vi "Hardware Manual Controller.vi"(6 "Simulated":bool, 7 "Simulated Actual Pressure":dbl, 8 "error in (no error)":errorcluster, 9 "Manual Control Cluster":T1 {"Speed" scale=0.0..10.0}, 10 "DAQ Ref Cluster in":T4, 11 "State Machine Data":T2={"Control State"="", "Status Message"="", "Speed"=0.0, "Pressure"=0.0, "Target Pressure"=0.0, "Apply Brake Ref"=refnum, "Release Brake Ref"=refnum, "Extend Ref"=refnum, "Retract Ref"=refnum, "Pressure Ref"=refnum, "Data Display Ref"=refnum, "Exit Button Ref"=refnum, "Bool"=TRUE, "Status"={"Extend"=FALSE, "Brake"=FALSE, "Retract"=FALSE}}) -> (0 "error out":errorcluster, 2 "DAQ Ref Cluster out":T4, 3 "Data Cluster out":T5)   [LabVIEW 2021]
uses:
  Controls/UI Data.ctl
  Controls/Status Lights.ctl
  Controls/DAQ Refnums.ctl
  Controls/State Machine Data.ctl
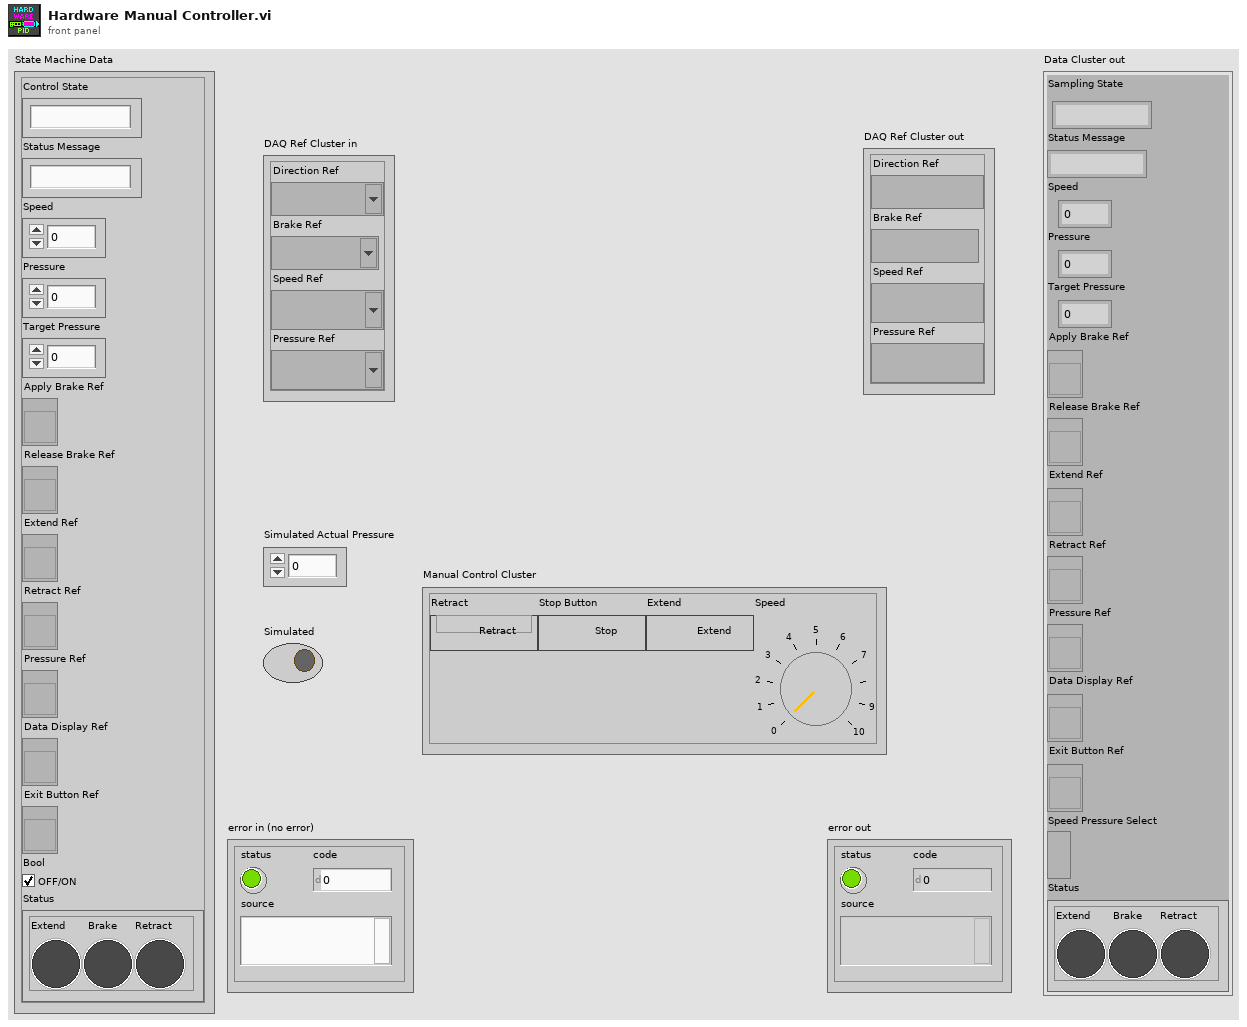
[diagram p1: front panel]
types:
  T1 = cluster{"Retract":bool, "Stop Button":bool, "Extend":bool, "Speed":dbl}
  T2 = typedef "State Machine Data.ctl" = cluster{"Control State":string, "Status Message":string, "Speed":dbl, "Pressure":dbl, "Target Pressure":dbl, "Apply Brake Ref":refnum<vi>, "Release Brake Ref":refnum<vi>, "Extend Ref":refnum<vi>, "Retract Ref":refnum<vi>, "Pressure Ref":refnum<vi>, "Data Display Ref":refnum<vi>, "Exit Button Ref":refnum<vi>, "Bool":bool, "Status":T3}
  T3 = typedef "Status Lights.ctl" = cluster{"Extend":bool, "Brake":bool, "Retract":bool}
  T4 = typedef "DAQ Refnums.ctl" = cluster{"Direction Ref":refnum<k21>, "Brake Ref":refnum<k21>, "Speed Ref":refnum<k21>, "Pressure Ref":refnum<k21>}
  T5 = typedef "UI Data.ctl" = cluster{"Sampling State":string, "Status Message":string, "Speed":dbl, "Pressure":dbl, "Target Pressure":dbl, "Apply Brake Ref":refnum<vi>, "Release Brake Ref":refnum<vi>, "Extend Ref":refnum<vi>, "Retract Ref":refnum<vi>, "Pressure Ref":refnum<vi>, "Data Display Ref":refnum<vi>, "Exit Button Ref":refnum<vi>, "Speed Pressure Select":bool, "Status":T3}
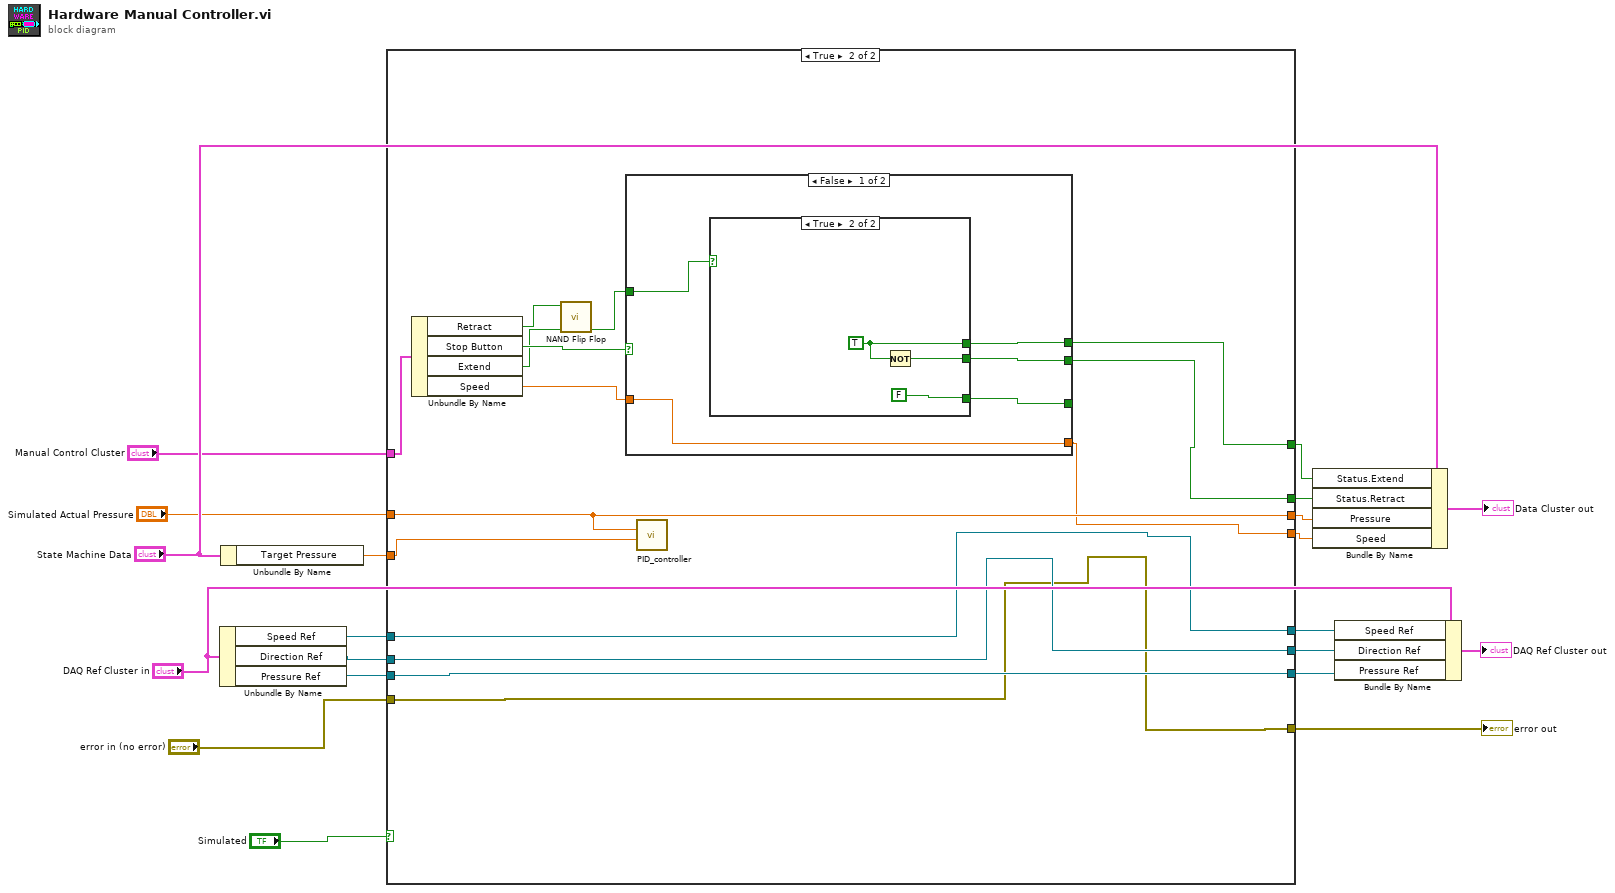
[diagram p0: block diagram]
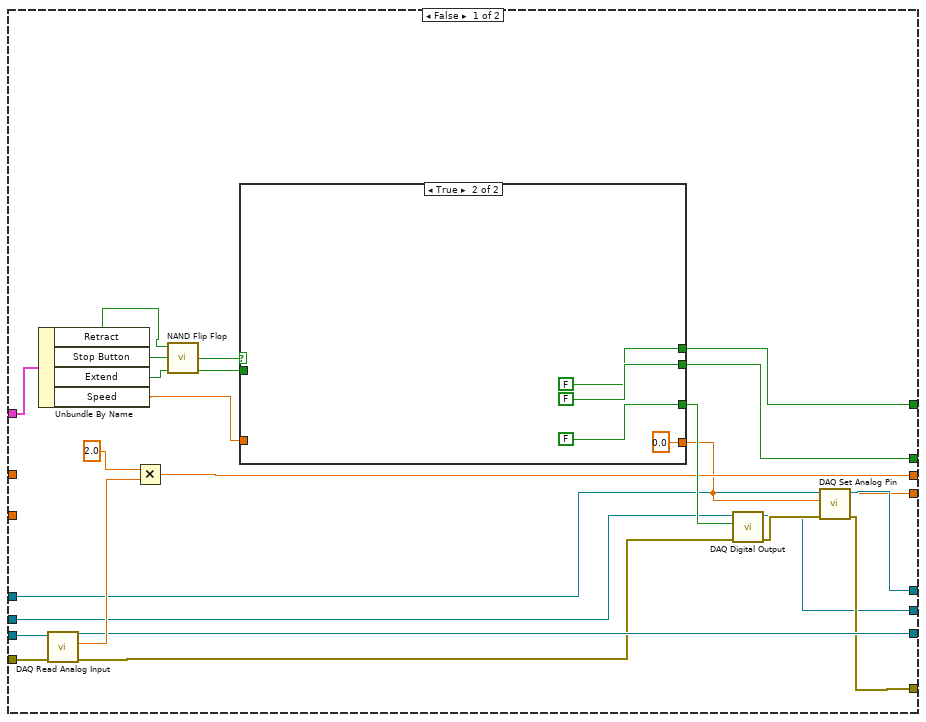
[diagram p2: hidden frame]
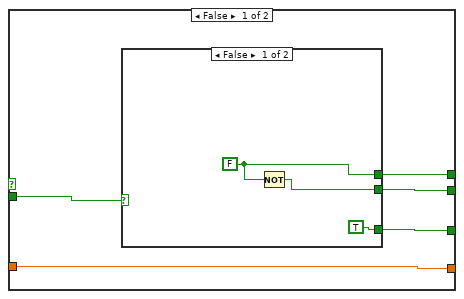
[diagram p3: hidden frame]
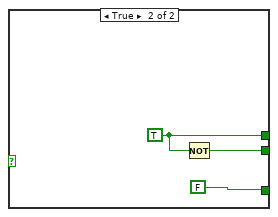
[diagram p4: hidden frame]
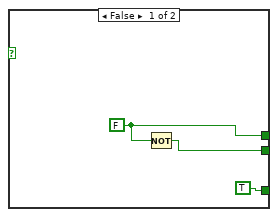
[diagram p5: hidden frame]
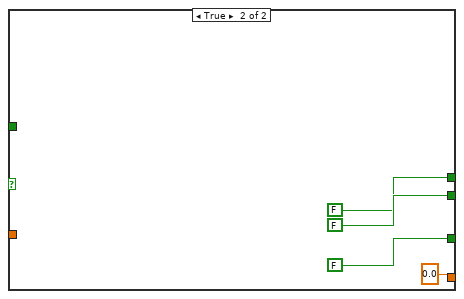
[diagram p6: hidden frame]
diagram:
  n1 = Unbundle By Name("DAQ Ref Cluster in") -> ("Speed Ref"=w10:refnum<k21>, "Direction Ref"=w12:refnum<k21>, "Pressure Ref"=w14:refnum<k21>)
  n2 = Unbundle By Name("State Machine Data") -> ("Target Pressure"=w20:dbl)
  n3 = case shown="True" "Simulated" {
    tunnel: w20 -> [_ w73]
    tunnel: "error in (no error)" -> [w43 w68]
    tunnel: [w41 w72] -> w18
    tunnel: w14 -> [w40 w72]
    tunnel: [w36 w68] -> w13
    tunnel: w12 -> [w35 w70]
    tunnel: [w34 w70] -> w11
    tunnel: w10 -> [w33 w69]
    tunnel: [w32 w69] -> w9
    tunnel: [w21 w61] -> w8
    tunnel: [w28 w71] -> w7
    tunnel: [w30 w67] -> w5
    tunnel: [w29 w66] -> w4
    tunnel: "Simulated Actual Pressure" -> [_ w71]
    tunnel: "Manual Control Cluster" -> [w27 w64]
    frame False {
      n4 = Unbundle By Name(w27) -> ("Retract"=w24:bool, "Stop Button"=w26:bool, "Extend"=w25:bool, "Speed"=w22:dbl)
      n5 = call "DAQ Read Analog Input.vi"("error in"=w43, "task/channels in"=w40) -> ("error out"=w38:errorcluster, "Voltage"=w42:dbl, "task out"=w41:refnum<k21>)  [unwired: 7 in]
      n6 = Multiply(x=2.0, y=w42) -> (x*y=w28:dbl)
      n7 = call "NAND Flip Flop.vi"("Reset"=w25, "Set"=w24) -> ("!Q"=w23:bool)  [unwired: 8 in, 1 out]
      n8 = case shown="True" w26 {
        tunnel: [w48 FALSE ("data")] -> w39
        tunnel: [w47 FALSE ("Status.Extend")] -> w30
        tunnel: [w46 FALSE] -> w29
        tunnel: w23 -> [w45 _]
        tunnel: [w44 0.0 ("Speed")] -> w21
        tunnel: w22 -> [w44 _]
        frame False {
          n9 = case shown="False" w45 {
            tunnel: [TRUE ("data") FALSE ("data")] -> w48
            tunnel: [w49 w54] -> w47
            tunnel: [w50 w53] -> w46
            frame False {
              w49 = FALSE ("Status.Extend")
              n10 = Not(x=w49) -> (.not. x?=w50:bool)
            }
            frame True {
              w54 = TRUE ("Status.Extend")
              n11 = Not(x=w54) -> (.not. x?=w53:bool)
            }
          }
        }
        frame True {
        }
      }
      n12 = call "DAQ Digital Output.vi"("error in"=w38, "data"=w39, "task/channels in"=w35) -> ("error out"=w37:errorcluster, "task out"=w34:refnum<k21>)  [unwired: 6 in, 1 out]
      n13 = call "DAQ Set Analog Pin.vi"("error in"=w37, "Voltage"=w21, "task/channels in"=w33) -> ("error out"=w36:errorcluster, "task out"=w32:refnum<k21>)  [unwired: 6 in, 1 out]
    }
    frame True {
      n14 = Unbundle By Name(w64) -> ("Retract"=w63:bool, "Stop Button"=w65:bool, "Extend"=w62:bool, "Speed"=w60:dbl)
      n15 = call "NAND Flip Flop.vi"("Reset"=w62, "Set"=w63) -> ("!Q"=w59:bool)  [unwired: 8 in, 1 out]
      n16 = case shown="False" w65 {
        tunnel: [w78 FALSE ("data")] -> _
        tunnel: [w77 FALSE ("Status.Extend")] -> w67
        tunnel: [w76 FALSE] -> w66
        tunnel: w59 -> [w75 _]
        tunnel: [w74 0.0 ("Speed")] -> w61
        tunnel: w60 -> [w74 _]
        frame False {
          n17 = case shown="True" w75 {
            tunnel: [TRUE ("data") FALSE ("data")] -> w78
            tunnel: [w79 w84] -> w77
            tunnel: [w80 w83] -> w76
            frame False {
              w79 = FALSE ("Status.Extend")
              n18 = Not(x=w79) -> (.not. x?=w80:bool)
            }
            frame True {
              w84 = TRUE ("Status.Extend")
              n19 = Not(x=w84) -> (.not. x?=w83:bool)
            }
          }
        }
        frame True {
        }
      }
      n20 = call "PID_controller.vi"("Setpoint"=w73, "Process Variable"=w71) -> ()  [unwired: 6 in, 4 out]
    }
  }
  "error out" <- w13
  n21 = Bundle By Name(cluster="State Machine Data", "Status.Extend"=w5, "Status.Retract"=w4, "Pressure"=w7, "Speed"=w8) -> (→"Data Cluster out":T2)
  n22 = Bundle By Name(cluster="DAQ Ref Cluster in", "Speed Ref"=w9, "Direction Ref"=w11, "Pressure Ref"=w18) -> (→"DAQ Ref Cluster out":T4)
